vi "Write Get Meta Data.vi"(8 "error in":errorcluster, 10 "Get Meta Data":T1, 11 "VISA Interface in":refnum<class "VISA Interface.lvclass">) -> (0 "error out":errorcluster, 3 "VISA Interface out":refnum<class "VISA Interface.lvclass">)   [LabVIEW 2020, in "Plugin Instrument Driver.lvlib" / "VISA Interface.lvclass"]
doc: "Get Meta Data"
uses:
  VISA Interface.lvclass
  builds/Libraries/Shared GUI Library.lvlibp/Shared GUI Library/Device Meta Data Cluster/Get Meta Data.ctl
  VISA Interface.lvclass/VISA Interface.ctl
  builds/Libraries/Shared GUI Library.lvlibp
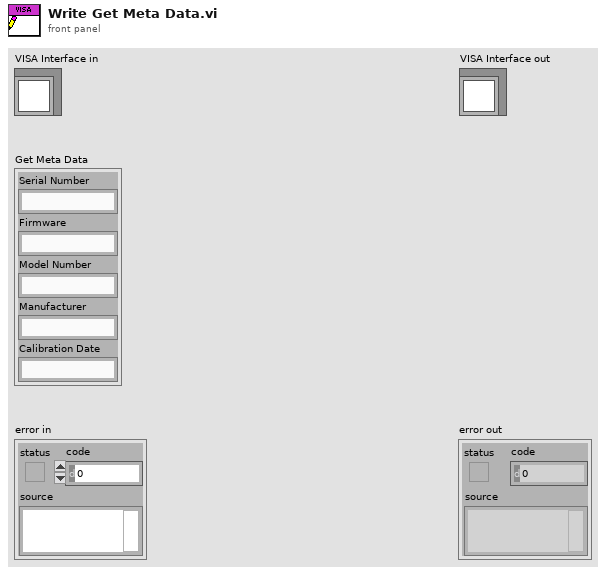
[diagram p1: front panel]
types:
  T1 = typedef "Shared GUI Library.lvlibp/Get Meta Data.ctl" = cluster{"Serial Number":string, "Firmware":string, "Model Number":string, "Manufacturer":string, "Calibration Date":string}
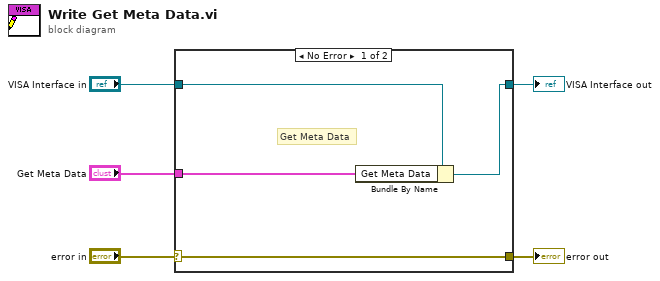
[diagram p0: block diagram]
diagram:
  n1 = case shown="No Error" "error in" {
    selector: "error in" -> [w9 w10]
    tunnel: [w9 w10] -> w4
    tunnel: [w7 w11] -> w2
    tunnel: "VISA Interface in" -> [w8 w11]
    tunnel: "Get Meta Data" -> [w6 _]
    frame No Error {
      # "Get Meta Data"
      n2 = Bundle By Name(cluster=w8, "Get Meta Data"=w6) -> (w7:refnum<class "VISA Interface.lvclass">)
    }
    frame Error {
    }
  }
  "error out" <- w4
  "VISA Interface out" <- w2
